vi "LabelGlobal.vi"(6 "New Element":cluster{"Address":i32, "Checksum":u32}, 7 "Add":bool) -> (2 "Lookup Table":cluster{"Address":i32, "Checksum":u32}[](array[cluster]))   [LabVIEW 2012, in "CRef.lvlib"]
uses:
  CRef.lvlib
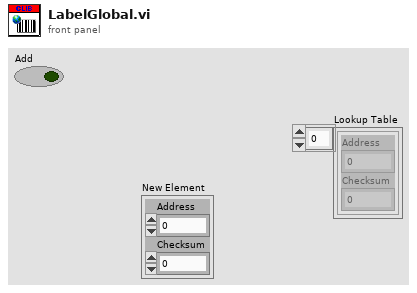
[diagram p1: front panel]
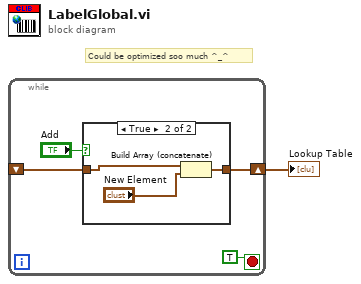
[diagram p0: block diagram]
diagram:
  # "Could be optimized soo much ^_^"
  n1 = while {
    shift-right: [w2] -> w1
    shift-left: _ -> [w4]
    stop <- TRUE stop-if-true
    n2 = case shown="True" "Add" {
      tunnel: w4 -> [w6 w9]
      tunnel: [w6 w8] -> w2
      frame False {
      }
      frame True {
        n3 = Build Array (concatenate)(w9, "New Element") -> (w8:cluster{"Address":i32, "Checksum":u32}[])
      }
    }
  }
  "Lookup Table" <- w1
